vi "HW_Init.vi"(8 "error in":errorcluster, 9 "Traget FPS":i32=80, 10 "Close port? (T)":bool=TRUE, 11 "VISA resource name":refnum<visa-resource-name>="Tracker") -> (0 "error out":errorcluster, 1 "Sensors response":string, 2 "Instrument OK?":bool=TRUE, 3 "VISA resource name out":refnum<visa-resource-name>="ASRL3::INSTR", 4 "Sync mode status":string, 5 "Sensor board size":string, 6 "FPS status":i32=80, 7 "Version information":string)   [LabVIEW 2018, in "Tracker.lvlib"]
uses:
  Tracker.lvlib
  <vilib>/Utility/error.llb/DialogType.ctl
  <vilib>/Instr/_visa.llb/VISA Set IO Buffer Mask.ctl
  <vilib>/Instr/_visa.llb/VISA Flush IO Buffer Mask.ctl
  <vilib>/Instr/_visa.llb/VISA Configure Serial Port (Instr).vi
panel:
  out "Poll Sync mode status":u32
  out "Poll Port data status":u32
  out "Port data status":i32=1
  out "Latest Poll results (before implemented adjustments)":string="P\r\nI am alive!\r\nA1454 OK!\r\nBinary mode ON\r\nCoordinate mode ON\r\nMatrix mode OFF\r\nFPS target=80\r\nExternal USART status: 0\r\nLed status: 1\r\nPort data status: 1\r\nIOS: 1 = 0, 2 = 0 3 = 0, 4 = 0\r\nOK\r\n"
  out "Poll Binary":u32
  out "Poll Matrix":u32
  out "Poll Coord":u32
  out "Poll FPS":u32
  out "Matrix mode status":string="OFF"
  out "Coordinate mode status":string="ON"
  out "Binary mode status":string="ON"
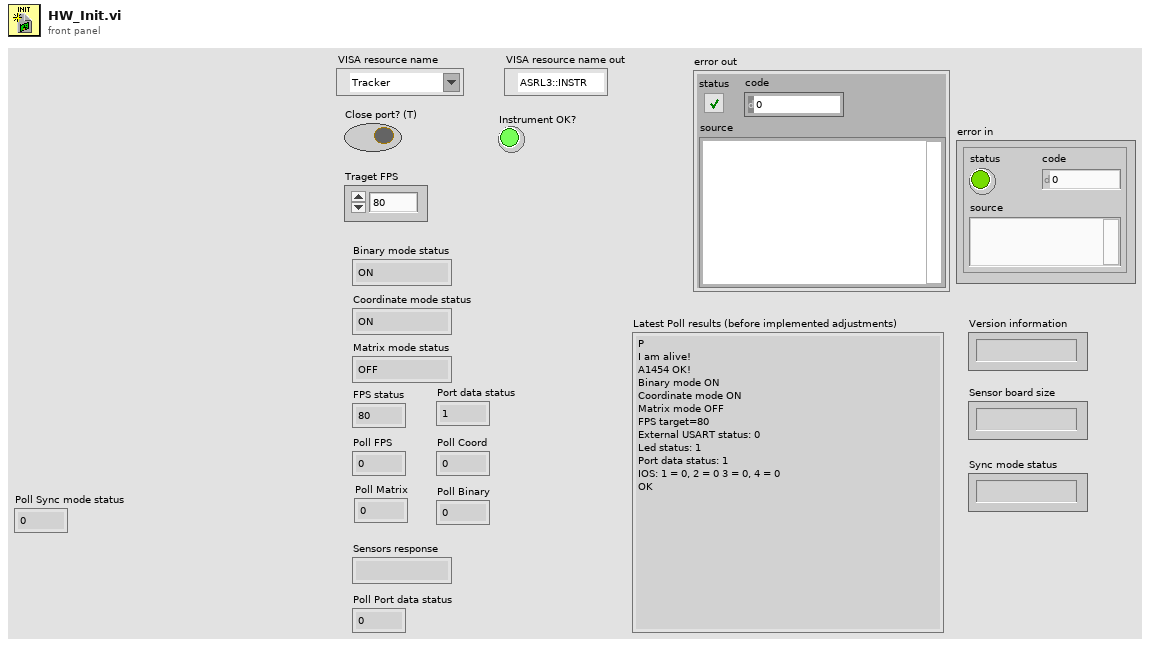
[diagram p1: front panel]
types:
  T1 = typedef "DialogType.ctl" = u16
  T2 = typedef "VISA Set IO Buffer Mask.ctl" = u16
  T3 = typedef "VISA Flush IO Buffer Mask.ctl" = u16
  T4 = cluster{"Matrix mode status":string, "Coordinate mode status":string, "Binary mode status":string, "Sensors response":string, "FPS status":i32, "Port data status":i32}
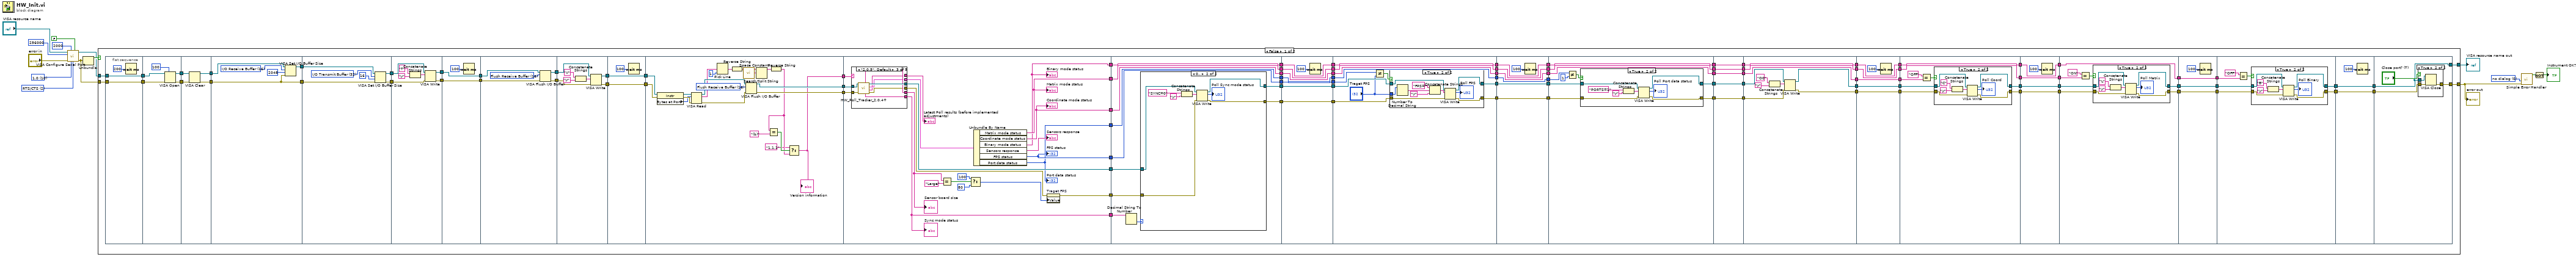
[diagram p0: block diagram]
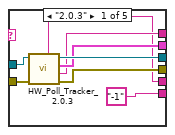
[diagram p2: hidden frame]
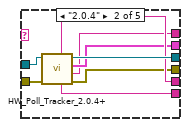
[diagram p3: hidden frame]
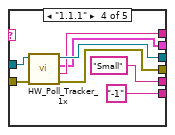
[diagram p4: hidden frame]
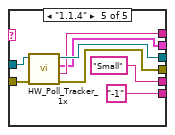
[diagram p5: hidden frame]
diagram:
  w1 = u16 10 items=["1.0"=10, "1.5"=15, "2.0"=20] ("stop bits (10: 1 bit)")
  w3 = T1 0 items=["no dialog", "OK message", "continue or stop message", "OK message + warnings", "continue/stop + warnings"] ("type of dialog (OK msg:1)")
  w9 = u16 2 items=["None", "XON/XOFF", "RTS/CTS", "XON/XOFF & RTS/CTS", "DTR/DSR", "XON/XOFF & DTR/DSR"] ("flow control (0:none)")
  n1 = call-poly "VISA Configure Serial Port"("VISA resource name"="VISA resource name", "timeout (10sec)"=u32 2000, "Enable Termination\nChar (T)"=FALSE ("Enable Termination\nChar (T)"), "baud rate (9600)"=u32 256000, "error in (no error)"="error in", "stop bits (10: 1 bit)"=w1, "flow control (0:none)"=w9) -> ("VISA resource name out"=w7:refnum<visa-resource-name>, "error out"=w11:errorcluster)  [unwired: 7 in]
  n2 = Unbundle(w11) -> ("status"=w10:bool)  [unwired: 2 out]
  n3 = case shown="False" w10 {
    tunnel: w7 -> [w83 w419]
    tunnel: w11 -> [w82 w420]
    tunnel: [w69 w420] -> w6
    tunnel: [w68 w419] -> w8
    frame False {
      n4 = flat-sequence {
        tunnel: [w116] -> w114
        tunnel: [w115] -> w113
        tunnel: w83 -> [w116]
        tunnel: w82 -> [w115]
        tunnel: w114 -> [w120]
        tunnel: [w119] -> w111
        tunnel: w113 -> [w122]
        tunnel: [w121] -> w112
        tunnel: w112 -> [w125]
        tunnel: w111 -> [w126]
        tunnel: [w124] -> w110
        tunnel: [w123] -> w109
        tunnel: [w127] -> w107
        tunnel: [w131] -> w108
        tunnel: w110 -> [w127]
        tunnel: w109 -> [w129]
        tunnel: w108 -> [w135]
        tunnel: [w134] -> w61
        tunnel: w107 -> [w133]
        tunnel: [w132] -> w60
        tunnel: w61 -> [w141]
        tunnel: [w139] -> w57
        tunnel: w60 -> [w140]
        tunnel: [w138] -> w55
        tunnel: w57 -> [w147]
        tunnel: [w147] -> w56
        tunnel: w55 -> [w146]
        tunnel: [w146] -> w54
        tunnel: w56 -> [w150]
        tunnel: [w149] -> w59
        tunnel: w54 -> [w152]
        tunnel: [w151] -> w58
        tunnel: w59 -> [w155]
        tunnel: w58 -> [w156]
        tunnel: [w154] -> w67
        tunnel: [w153] -> w66
        tunnel: w67 -> [w162]
        tunnel: [w162] -> w65
        tunnel: w66 -> [w161]
        tunnel: [w161] -> w63
        tunnel: w65 -> [w179]
        tunnel: [w177] -> w64
        tunnel: w63 -> [w180]
        tunnel: [w175] -> w62
        tunnel: [w164] -> w53
        tunnel: [w191] -> w44
        tunnel: [w204] -> w45
        tunnel: w64 -> [w202]
        tunnel: [w195] -> w42
        tunnel: [w198] -> w40
        tunnel: [w199] -> w38
        tunnel: [w197] -> w36
        tunnel: [w194] -> w34
        tunnel: w62 -> [w201]
        tunnel: w53 -> [w193]
        tunnel: [w184] -> w31
        tunnel: w45 -> [w250]
        tunnel: w44 -> [w248]
        tunnel: [w247] -> w43
        tunnel: w42 -> [w255]
        tunnel: [w255] -> w41
        tunnel: w40 -> [w254]
        tunnel: [w254] -> w39
        tunnel: w38 -> [w253]
        tunnel: [w253] -> w37
        tunnel: w36 -> [w252]
        tunnel: [w252] -> w35
        tunnel: w34 -> [w251]
        tunnel: [w251] -> w33
        tunnel: [w249] -> w32
        tunnel: w31 -> [w246]
        tunnel: [w273] -> w52
        tunnel: w43 -> [w272]
        tunnel: [w272] -> w51
        tunnel: w41 -> [w271]
        tunnel: [w271] -> w50
        tunnel: w39 -> [w270]
        tunnel: [w270] -> w49
        tunnel: w37 -> [w269]
        tunnel: [w269] -> w48
        tunnel: w35 -> [w268]
        tunnel: [w268] -> w47
        tunnel: w33 -> [w267]
        tunnel: [w267] -> w46
        tunnel: w32 -> [w273]
        tunnel: w52 -> [w282]
        tunnel: [w279] -> w106
        tunnel: w51 -> [w281]
        tunnel: [w280] -> w105
        tunnel: w50 -> [w283]
        tunnel: [w278] -> w104
        tunnel: w49 -> [w278]
        tunnel: [w277] -> w103
        tunnel: w48 -> [w277]
        tunnel: [w276] -> w102
        tunnel: w47 -> [w276]
        tunnel: w46 -> [w275]
        tunnel: [w275] -> w70
        tunnel: w106 -> [w303]
        tunnel: [w303] -> w81
        tunnel: w105 -> [w302]
        tunnel: [w302] -> w80
        tunnel: [w300] -> w79
        tunnel: w104 -> [w300]
        tunnel: [w299] -> w78
        tunnel: w103 -> [w299]
        tunnel: [w298] -> w77
        tunnel: w102 -> [w298]
        tunnel: [w297] -> w71
        tunnel: w70 -> [w297]
        tunnel: w81 -> [w308]
        tunnel: [w307] -> w76
        tunnel: w80 -> [w310]
        tunnel: [w309] -> w75
        tunnel: w79 -> [w313]
        tunnel: [w313] -> w74
        tunnel: w78 -> [w312]
        tunnel: [w312] -> w73
        tunnel: w77 -> [w311]
        tunnel: [w311] -> w72
        tunnel: w71 -> [w305]
        tunnel: w76 -> [w328]
        tunnel: [w328] -> w30
        tunnel: w75 -> [w327]
        tunnel: [w327] -> w29
        tunnel: w74 -> [w326]
        tunnel: [w326] -> w28
        tunnel: w73 -> [w325]
        tunnel: [w325] -> w27
        tunnel: w72 -> [w324]
        tunnel: [w324] -> w26
        tunnel: w30 -> [w332]
        tunnel: [w331] -> w25
        tunnel: w29 -> [w330]
        tunnel: [w329] -> w23
        tunnel: w28 -> [w338]
        tunnel: [w338] -> w21
        tunnel: w27 -> [w337]
        tunnel: [w337] -> w19
        tunnel: w26 -> [w336]
        tunnel: [w336] -> w17
        tunnel: w25 -> [w344]
        tunnel: [w344] -> w24
        tunnel: w23 -> [w343]
        tunnel: [w343] -> w22
        tunnel: w21 -> [w342]
        tunnel: [w342] -> w20
        tunnel: w19 -> [w341]
        tunnel: [w341] -> w18
        tunnel: w17 -> [w340]
        tunnel: [w340] -> w16
        tunnel: w24 -> [w352]
        tunnel: [w350] -> w101
        tunnel: w22 -> [w351]
        tunnel: [w347] -> w100
        tunnel: w20 -> [w349]
        tunnel: w18 -> [w346]
        tunnel: [w346] -> w99
        tunnel: w16 -> [w345]
        tunnel: [w345] -> w98
        tunnel: w101 -> [w368]
        tunnel: [w368] -> w97
        tunnel: w100 -> [w367]
        tunnel: [w367] -> w96
        tunnel: [w365] -> w95
        tunnel: w99 -> [w365]
        tunnel: [w364] -> w94
        tunnel: w98 -> [w364]
        tunnel: w97 -> [w374]
        tunnel: [w372] -> w93
        tunnel: w96 -> [w373]
        tunnel: [w371] -> w92
        tunnel: w95 -> [w370]
        tunnel: w94 -> [w369]
        tunnel: [w369] -> w91
        tunnel: w93 -> [w390]
        tunnel: [w390] -> w90
        tunnel: w92 -> [w389]
        tunnel: [w389] -> w89
        tunnel: [w387] -> w88
        tunnel: w91 -> [w387]
        tunnel: w90 -> [w395]
        tunnel: [w393] -> w87
        tunnel: w89 -> [w394]
        tunnel: [w392] -> w86
        tunnel: w88 -> [w391]
        tunnel: w87 -> [w410]
        tunnel: [w410] -> w85
        tunnel: [w409] -> w84
        tunnel: w86 -> [w409]
        tunnel: w85 -> [w411]
        tunnel: w84 -> [w414]
        tunnel: [w412] -> w69
        tunnel: [w411] -> w68
        frame #0 {
          n5 = Wait (ms)(milliseconds to wait=u32 200) -> ()  [unwired: 1 out]
        }
        frame #1 {
          n6 = VISA Open(timeout (0)=u32 100 ("VISA Open timeout (0)"), error in (no error)=w122, VISA resource name=w120) -> (VISA resource name=w119:refnum<visa-resource-name>, error out=w121:errorcluster)  [unwired: 2 in]
        }
        frame #2 {
          n7 = VISA Clear(VISA resource name=w126, error in (no error)=w125) -> (VISA resource name out=w123:refnum<visa-resource-name>, error out=w124:errorcluster)
        }
        frame #3 {
          w128 = T2 16 items=["I/O Receive Buffer"=16, "I/O Transmit Buffer"=32, "I/O Receive and Transmit Buffer"=48] ("Mask")
          n8 = VISA Set I/O Buffer Size(VISA resource name=w129, mask (16)=w128, size (4096)=u32 2048, error in (no error)=w127) -> (VISA resource name out=w131:refnum<visa-resource-name>)  [unwired: 1 out]
        }
        frame #4 {
          w136 = T2 32 items=["I/O Receive Buffer"=16, "I/O Transmit Buffer"=32, "I/O Receive and Transmit Buffer"=48] ("Mask")
          n9 = VISA Set I/O Buffer Size(VISA resource name=w135, mask (16)=w136, size (4096)=u32 16, error in (no error)=w133) -> (VISA resource name out=w134:refnum<visa-resource-name>, error out=w132:errorcluster)
        }
        frame #5 {
          n10 = Concatenate Strings("T" ("write buffer"), "\r") -> (w142:string)
          n11 = VISA Write(VISA resource name=w141, write buffer=w142, error in (no error)=w140) -> (VISA resource name out=w139:refnum<visa-resource-name>, error out=w138:errorcluster)  [unwired: 1 out]
        }
        frame #6 {
          n12 = Wait (ms)(milliseconds to wait=u32 100) -> ()  [unwired: 1 out]
        }
        frame #7 {
          w148 = T3 16 items=["Flush Receive Buffer"=16, "Write Transmit Buffer to Device"=32, "Flush Receive Buffer (No I/O)"=64, "Flush Transmit Buffer"=128] ("Mask")
          n13 = VISA Flush I/O Buffer(VISA resource name=w150, mask (16)=w148, error in (no error)=w152) -> (VISA resource name out=w149:refnum<visa-resource-name>, error out=w151:errorcluster)
        }
        frame #8 {
          n14 = Concatenate Strings("V" ("write buffer"), "\r") -> (w157:string)
          n15 = VISA Write(VISA resource name=w155, write buffer=w157, error in (no error)=w156) -> (VISA resource name out=w153:refnum<visa-resource-name>, error out=w154:errorcluster)  [unwired: 1 out]
        }
        frame #9 {
          n16 = Wait (ms)(milliseconds to wait=u32 100) -> ()  [unwired: 1 out]
        }
        frame #10 {
          w174 = T3 16 items=["Flush Receive Buffer"=16, "Write Transmit Buffer to Device"=32, "Flush Receive Buffer (No I/O)"=64, "Flush Transmit Buffer"=128] ("Mask")
          n17 = property class="Instr"(reference=w180, error in=w179) -> (reference out=w183:refnum<visa-resource-name>, error out=w182:errorcluster, "Bytes at Port"=w181:u32)
          n18 = VISA Read(VISA resource name=w183, byte count=w181, error in (no error)=w182) -> (VISA resource name out=w176:refnum<visa-resource-name>, read buffer=w173:string, error out=w178:errorcluster)  [unwired: 1 out]
          n19 = Pick Line(multi-line string=w173, line index=1) -> (output string=w171:string)  [unwired: 1 in]
          n20 = Reverse String(1:w171) -> (0:w170:string)
          n21 = call <vilib>:"Space Constant.vi"() -> ("String"=w169:string)
          n22 = VISA Flush I/O Buffer(VISA resource name=w176, mask (16)=w174, error in (no error)=w178) -> (VISA resource name out=w175:refnum<visa-resource-name>, error out=w177:errorcluster)
          n23 = Search/Split String(string=w170, search string/char (-)=w169) -> (substring before match=w168:string)  [unwired: 1 in, 2 out]
          n24 = Reverse String(1:w168) -> (0:w165:string)
          n25 = Equal?(x=w165, y="(b)") -> (x = y?=w166:bool)
          n26 = Select(t="1.1.1", s=w166, f=w165) -> (s? t:f=w164:string)
          "Version information" <- w164
        }
        frame #11 {
          n27 = case shown="\"2.0.5\", Default" w193 {
            tunnel: [w209 w218 w226 w236 w244] -> w204
            tunnel: [w207 w215 w223 w235 w243] -> w203
            tunnel: w202 -> [w212 w219 w227 w234 w242]
            tunnel: w201 -> [w210 w220 w228 w233 w241]
            tunnel: [w211 w214 w222 w232 w240] -> w192
            tunnel: [w208 w216 w224 w231 w239] -> w200
            tunnel: [w206 w217 w225 "Small" "Small"] -> w190
            tunnel: ["-1" ("Sync mode status") w213 w221 "-1" ("Sync mode status") "-1" ("Sync mode status")] -> w184
            frame "2.0.3" {
              n28 = call "HW_Poll_Tracker_2.0.3.vi"("error in"=w212, "VISA resource name in"=w210) -> ("error out"=w211:errorcluster, "Read buffer"=w207:string, "Parameters output"=w208:T4, "VISA resource name out"=w209:refnum<visa-resource-name>, "Sensor board size"=w206:string)  [unwired: 5 in]
            }
            frame "2.0.4" {
              n29 = call "HW_Poll_Tracker_2.0.4+.vi"("error in"=w219, "VISA resource name in"=w220) -> ("error out"=w214:errorcluster, "Read buffer"=w215:string, "Parameters output"=w216:T4, "VISA resource name out"=w218:refnum<visa-resource-name>, "Sync mode status"=w213:string, "Sensor board size"=w217:string)  [unwired: 4 in]
            }
            frame "2.0.5", Default {
              n30 = call "HW_Poll_Tracker_2.0.4+.vi"("error in"=w227, "VISA resource name in"=w228) -> ("error out"=w222:errorcluster, "Read buffer"=w223:string, "Parameters output"=w224:T4, "VISA resource name out"=w226:refnum<visa-resource-name>, "Sync mode status"=w221:string, "Sensor board size"=w225:string)  [unwired: 4 in]
            }
            frame "1.1.1" {
              n31 = call "HW_Poll_Tracker_1x.vi"("error in"=w234, "VISA resource name in"=w233) -> ("error out"=w232:errorcluster, "Read buffer"=w235:string, "Parameters output"=w231:T4, "VISA resource name out"=w236:refnum<visa-resource-name>)  [unwired: 6 in]
            }
            frame "1.1.4" {
              n32 = call "HW_Poll_Tracker_1x.vi"("error in"=w242, "VISA resource name in"=w241) -> ("error out"=w240:errorcluster, "Read buffer"=w243:string, "Parameters output"=w239:T4, "VISA resource name out"=w244:refnum<visa-resource-name>)  [unwired: 6 in]
            }
          }
          "Latest Poll results (before implemented adjustments)" <- w203
          "Sensor board size" <- w190
          "Sync mode status" <- w184
          n33 = Equal?(x=w190, y="Large") -> (x = y?=w188:bool)
          n34 = Select(t=100, s=w188, f=80) -> (s? t:f=w185:i32)
          n35 = Unbundle By Name(w200) -> ("Matrix mode status"=w199:string, "Coordinate mode status"=w198:string, "Binary mode status"=w197:string, "Sensors response"=→"Sensors response":string, "FPS status"=w195:i32, "Port data status"=w194:i32)
          "Binary mode status" <- w197
          "Coordinate mode status" <- w198
          "Matrix mode status" <- w199
          "FPS status" <- w195
          "Port data status" <- w194
          n36 = property on="Traget FPS" class="DigNum (strict)"(error in=w192, "Value"=w185) -> (error out=w191:errorcluster)  [unwired: 1 in, 1 out]
        }
        frame #12 {
          n37 = Decimal String To Number(string=w246) -> (number=w245:i32)  [unwired: 2 in, 1 out]
          n38 = case shown="0.." w245 {
            tunnel: w250 -> [w257 w263]
            tunnel: w248 -> [w256 w262]
            tunnel: [w256 w261] -> w247
            tunnel: [w257 w260] -> w249
            frame -1, Default {
            }
            frame 0.. {
              n39 = Concatenate Strings("SYNC=0" ("write buffer"), "\r") -> (w265:string)
              n40 = VISA Write(VISA resource name=w263, write buffer=w265, error in (no error)=w262) -> (VISA resource name out=w260:refnum<visa-resource-name>, return count=→"Poll Sync mode status":u32, error out=w261:errorcluster)
            }
          }
        }
        frame #13 {
          n41 = Wait (ms)(milliseconds to wait=u32 100) -> ()  [unwired: 1 out]
        }
        frame #14 {
          n42 = Not Equal?(x=w283, y="Traget FPS") -> (x != y?=w284:bool)
          n43 = case shown="True" w284 {
            tunnel: w282 -> [w286 w293]
            tunnel: w281 -> [w285 w292]
            tunnel: [w285 w291] -> w280
            tunnel: [w286 w290] -> w279
            tunnel: "Traget FPS" -> [_ w288]
            frame False {
            }
            frame True {
              n44 = Number To Decimal String(number=w288) -> (decimal integer string=w287:string)  [unwired: 1 in]
              n45 = Concatenate Strings("FPS=" ("write buffer"), w287, "\r") -> (w295:string)
              n46 = VISA Write(VISA resource name=w293, write buffer=w295, error in (no error)=w292) -> (VISA resource name out=w290:refnum<visa-resource-name>, return count=→"Poll FPS":u32, error out=w291:errorcluster)
            }
          }
        }
        frame #15 {
          n47 = Wait (ms)(milliseconds to wait=u32 100) -> ()  [unwired: 1 out]
        }
        frame #16 {
          n48 = Not Equal?(x=w305, y=1) -> (x != y?=w304:bool)
          n49 = case shown="True" w304 {
            tunnel: w310 -> [w314 w319]
            tunnel: [w314 w318] -> w309
            tunnel: w308 -> [w315 w317]
            tunnel: [w315 w316] -> w307
            frame False {
            }
            frame True {
              n50 = Concatenate Strings("PORTS=1" ("write buffer"), "\r") -> (w321:string)
              n51 = VISA Write(VISA resource name=w317, write buffer=w321, error in (no error)=w319) -> (VISA resource name out=w316:refnum<visa-resource-name>, return count=→"Poll Port data status":u32, error out=w318:errorcluster)
            }
          }
        }
        frame #17 {
        }
        frame #18 {
          n52 = Concatenate Strings("O0" ("write buffer"), "\r") -> (w333:string)
          n53 = VISA Write(VISA resource name=w332, write buffer=w333, error in (no error)=w330) -> (VISA resource name out=w331:refnum<visa-resource-name>, error out=w329:errorcluster)  [unwired: 1 out]
        }
        frame #19 {
          n54 = Wait (ms)(milliseconds to wait=u32 100) -> ()  [unwired: 1 out]
        }
        frame #20 {
          n55 = Equal?(x="OFF", y=w349) -> (x = y?=w353:bool)
          n56 = case shown="True" w353 {
            tunnel: w352 -> [w355 w359]
            tunnel: w351 -> [w354 w358]
            tunnel: [w355 w357] -> w350
            tunnel: [w354 w356] -> w347
            frame False {
            }
            frame True {
              n57 = Concatenate Strings("C" ("write buffer"), "\r") -> (w361:string)
              n58 = VISA Write(VISA resource name=w359, write buffer=w361, error in (no error)=w358) -> (VISA resource name out=w357:refnum<visa-resource-name>, return count=→"Poll Coord":u32, error out=w356:errorcluster)
            }
          }
        }
        frame #21 {
          n59 = Wait (ms)(milliseconds to wait=u32 100) -> ()  [unwired: 1 out]
        }
        frame #22 {
          n60 = Equal?(x="ON", y=w370) -> (x = y?=w376:bool)
          n61 = case shown="True" w376 {
            tunnel: w374 -> [w378 w382]
            tunnel: w373 -> [w377 w381]
            tunnel: [w378 w380] -> w372
            tunnel: [w377 w379] -> w371
            frame False {
            }
            frame True {
              n62 = Concatenate Strings("L" ("write buffer"), "\r") -> (w384:string)
              n63 = VISA Write(VISA resource name=w382, write buffer=w384, error in (no error)=w381) -> (VISA resource name out=w380:refnum<visa-resource-name>, return count=→"Poll Matrix":u32, error out=w379:errorcluster)
            }
          }
        }
        frame #23 {
          n64 = Wait (ms)(milliseconds to wait=u32 100) -> ()  [unwired: 1 out]
        }
        frame #24 {
          n65 = Equal?(x="OFF", y=w391) -> (x = y?=w397:bool)
          n66 = case shown="True" w397 {
            tunnel: w395 -> [w399 w403]
            tunnel: w394 -> [w398 w402]
            tunnel: [w399 w401] -> w393
            tunnel: [w398 w400] -> w392
            frame False {
            }
            frame True {
              n67 = Concatenate Strings("B" ("write buffer"), "\r") -> (w405:string)
              n68 = VISA Write(VISA resource name=w403, write buffer=w405, error in (no error)=w402) -> (VISA resource name out=w401:refnum<visa-resource-name>, return count=→"Poll Binary":u32, error out=w400:errorcluster)
            }
          }
        }
        frame #25 {
          n69 = Wait (ms)(milliseconds to wait=u32 100) -> ()  [unwired: 1 out]
        }
        frame #26 {
          n70 = case shown="True" "Close port? (T)" {
            tunnel: w414 -> [w415 w418]
            tunnel: [w415 w417] -> w412
            tunnel: w411 -> [_ w416]
            frame False {
            }
            frame True {
              n71 = VISA Close(VISA resource name=w416, error in (no error)=w418) -> (error out=w417:errorcluster)
            }
          }
        }
      }
    }
    frame True {
    }
  }
  "error out" <- w6
  "VISA resource name out" <- w8
  n72 = call <vilib>:"Simple Error Handler.vi"("type of dialog (OK msg:1)"=w3, "error in (no error)"=w6) -> ("error?"=w5:bool)  [unwired: 3 in, 4 out]
  n73 = Not(x=w5) -> (.not. x?=→"Instrument OK?":bool)
